vi "specRelay.vi"() -> (0 "RelaySpec":T1 {"Card Index" items=["Relay Card 1", "Relay Card 2", "Relay Card 3", "Relay Card 4", "Relay Card 5"]; "Relay Index" items=["Relay 1", "Relay 2", "Relay 3", "Relay 4", "Relay 5", "6", "7", "8", "9", "10", "11", "12"]})   [LabVIEW 2011]
uses:
  relaySpec.ctl
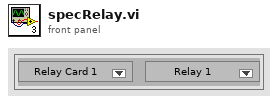
[diagram p1: front panel]
types:
  T1 = typedef "relaySpec.ctl" = cluster{"Card Index":u16, "Relay Index":u16}
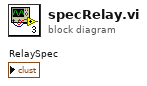
[diagram p0: block diagram]
diagram:
